vi "EvaluacionFinal.vi"(10 "Evaluacion Final":bool, 11 "Prueba32 in":refnum<class "Prueba32.lvclass">) -> ()   [LabVIEW 2019, in "Prueba32.lvclass"]
uses:
  Prueba32.lvclass
  Prueba32.lvclass/Prueba32.ctl
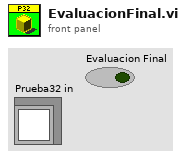
[diagram p1: front panel]
types:
  T1 = cluster{"ControlName":string, "ControlReference":refnum<vi>}[]
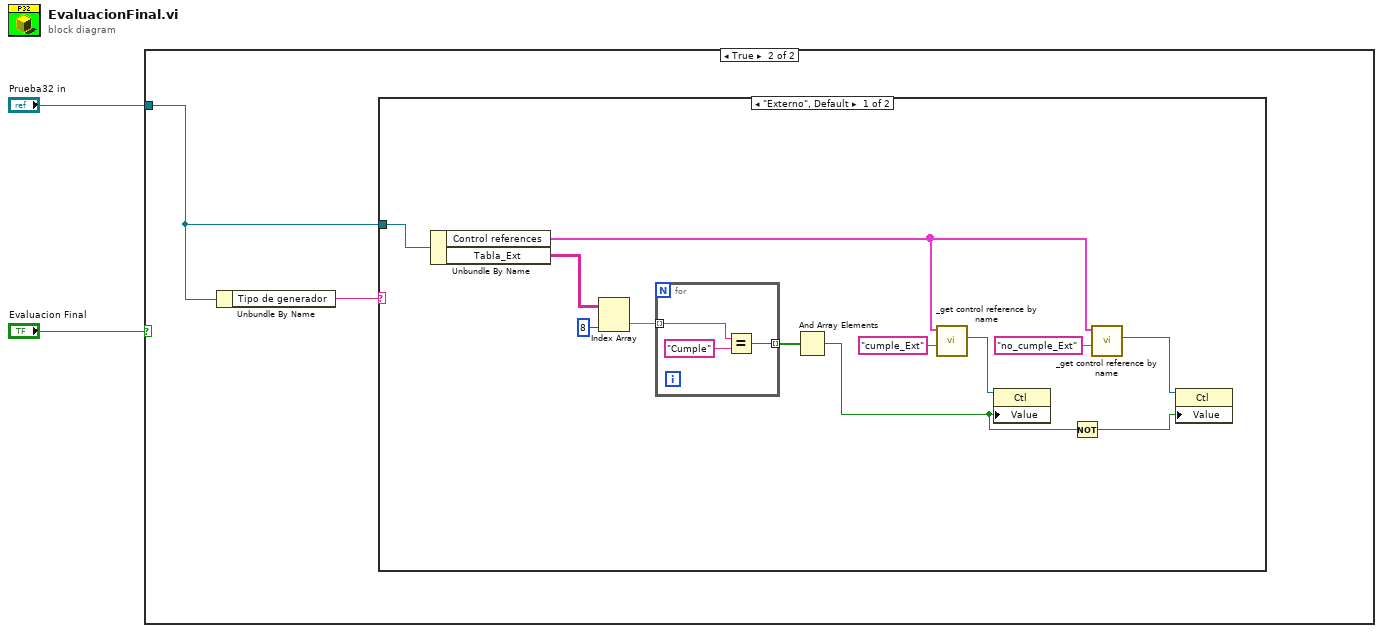
[diagram p0: block diagram]
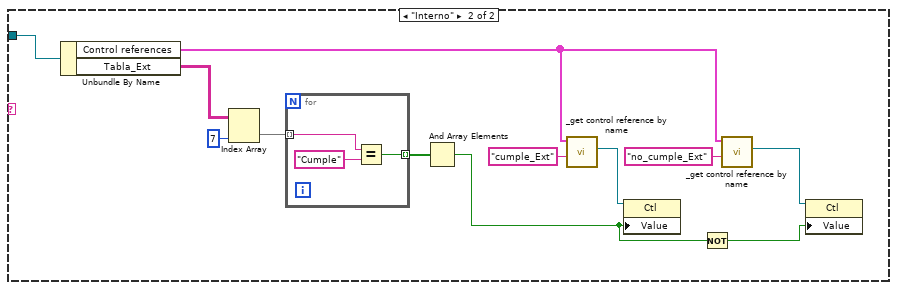
[diagram p3: hidden frame]
diagram:
  n1 = case shown="True" "Evaluacion Final" {
    tunnel: "Prueba32 in" -> [_ w3]
    frame False {
    }
    frame True {
      n2 = Unbundle By Name(w3) -> ("Tipo de generador"=w4:string)
      n3 = case shown="\"Externo\", Default" w4 {
        tunnel: w3 -> [w16 w31]
        frame "Externo", Default {
          n4 = Unbundle By Name(w16) -> ("Control references"=w8:T1, "Tabla_Ext"=w15:string[][])
          n5 = Index Array(array=w15, index (col)=8 ("disabled index (col)")) -> (element=w13:string[])  [unwired: 1 in]
          n6 = for {
            tunnel: w13 -> [w19] mode=indexing
            tunnel: [w17] -> w12 mode=indexing
            n7 = Equal?(x=w19, y="Cumple") -> (x = y?=w17:bool)
          }
          n8 = And Array Elements(Boolean array=w12) -> (logical AND=w6:bool)
          n9 = call "_get control reference by name.vi"("Control name"="cumple_Ext", "Control references"=w8) -> ("Ctl Refnum"=w10:refnum<vi>)  [unwired: 4 in, 1 out]
          n10 = property class="Ctl"(reference=w10, "Value"=w6) -> ()  [unwired: 1 in, 2 out]
          n11 = Not(x=w6) -> (.not. x?=w5:bool)
          n12 = call "_get control reference by name.vi"("Control name"="no_cumple_Ext", "Control references"=w8) -> ("Ctl Refnum"=w7:refnum<vi>)  [unwired: 4 in, 1 out]
          n13 = property class="Ctl"(reference=w7, "Value"=w5) -> ()  [unwired: 1 in, 2 out]
        }
        frame "Interno" {
          n14 = Unbundle By Name(w31) -> ("Control references"=w23:T1, "Tabla_Ext"=w30:string[][])
          n15 = Index Array(array=w30, index (col)=7 ("disabled index (col)")) -> (element=w28:string[])  [unwired: 1 in]
          n16 = for {
            tunnel: w28 -> [w34] mode=indexing
            tunnel: [w32] -> w27 mode=indexing
            n17 = Equal?(x=w34, y="Cumple") -> (x = y?=w32:bool)
          }
          n18 = And Array Elements(Boolean array=w27) -> (logical AND=w21:bool)
          n19 = call "_get control reference by name.vi"("Control name"="cumple_Ext", "Control references"=w23) -> ("Ctl Refnum"=w25:refnum<vi>)  [unwired: 4 in, 1 out]
          n20 = property class="Ctl"(reference=w25, "Value"=w21) -> ()  [unwired: 1 in, 2 out]
          n21 = Not(x=w21) -> (.not. x?=w20:bool)
          n22 = call "_get control reference by name.vi"("Control name"="no_cumple_Ext", "Control references"=w23) -> ("Ctl Refnum"=w22:refnum<vi>)  [unwired: 4 in, 1 out]
          n23 = property class="Ctl"(reference=w22, "Value"=w20) -> ()  [unwired: 1 in, 2 out]
        }
      }
    }
  }
